vi "EOL CAN_Start CAN.vi"(8 "error in (no error)":errorcluster, 11 "CAN Interface":refnum<k21>="CAN1") -> (0 "error out":errorcluster, 1 "Tester Write Session out":refnum<k21>, 2 "Read Session out":refnum<k21>, 3 "DSC Write Session out":refnum<k21>, 4 "time out session out":refnum<k21>)   [LabVIEW 2018]
uses:
  <vilib>/xnet/xnet.llb/XNET CAN Comm State.ctl
  <vilib>/xnet/xnet.llb/XNET Control Scope.ctl
  <vilib>/xnet/xnet.llb/XNET Frame CAN.ctl
  <vilib>/xnet/xnet.llb/XNET Frame Type CAN.ctl
  <vilib>/xnet/xnet.llb/XNET Create Session (Frame Input Queued).vi
  <vilib>/xnet/xnet.llb/XNET Create Session (Frame Output Single-point).vi
  <vilib>/xnet/xnet.llb/XNET Write (Frame CAN).vi
  <vilib>/xnet/xnet.llb/XNET Read (State CAN Comm).vi
  <vilib>/xnet/xnet.llb/XNET Wait (Interface Communicating).vi
  <resource>/objmgr/xnet.rc
panel:
  out "CAN:I/O Mode":u32(ring) items=["CAN 2.0", "CAN FD", "CAN FD+BRS"]
  out "Protocol":u32(ring) items=["CAN", "FlexRay", "LIN"]
  out "CAN:Transceiver Capability":u32(ring) items=["HS"=0, "LS"=1, "XS"=3, "XS (HS/LS)"=4]
  out "Interface:CAN:Transceiver State 3":u32(ring) items=["Normal", "Sleep", "Single Wire Wakeup", "Single Wire High-Speed"]
  out "Interface:CAN:Transceiver State 2":u32(ring) items=["Normal", "Sleep", "Single Wire Wakeup", "Single Wire High-Speed"]
  out "Interface:CAN:Transceiver State":u32(ring) items=["Normal", "Sleep", "Single Wire Wakeup", "Single Wire High-Speed"]
  out "PDUs":refnum<k21>[](array[refnum])
  out "Frames":refnum<k21>[](array[refnum])
  out "ECUs":refnum<k21>[](array[refnum])
  out "Database":refnum<k21>
  out "Configuration Status":i32
  out "CAN:Termination Capability":u32(ring) items=["No", "Yes"]
  out "Array":T1[](array[typedef]) items=["Error Active", "Error Passive", "Bus Off", "Init"]
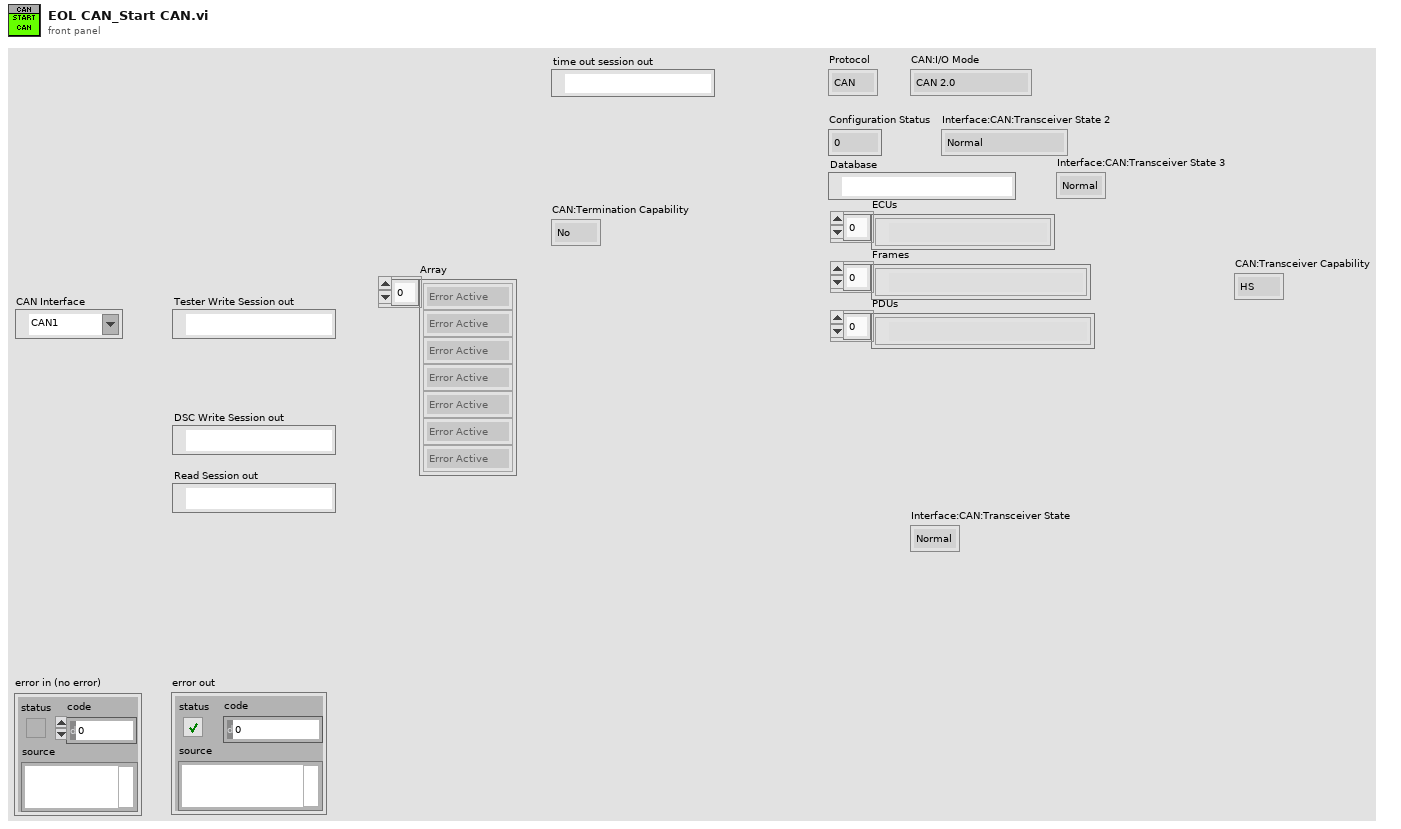
[diagram p1: front panel]
types:
  T1 = typedef "XNET CAN Comm State.ctl" = u8
  T2 = typedef "XNET Control Scope.ctl" = u32
  T3 = cluster{"Comment":string, "Default Payload":u8[], "Identifier":u32, "Name (Short)":string, "Payload Length":u32, "PDU_Mapping":cluster{"PDU":string, "Start Bit":u32, "Update Bit":i32}[], "CAN:Extended Identifier?":bool, "CAN:Timing Type":u32, "CAN:Transmit Time":dbl, "CAN:I/O Mode":u32}
  T4 = typedef "XNET Frame CAN.ctl" = cluster{"timestamp":timestamp, "payload":u8[], "identifier":u32, "type":T5, "extended?":bool, "echo?":bool}
  T5 = typedef "XNET Frame Type CAN.ctl" = u8
  T6 = typedef "XNET CAN Comm.ctl" = cluster{"fault code":i32, "fault?":bool, "communication state":T1, "last error":T7, "receive error counter":u8, "transmit error counter":u8, "transceiver error?":bool, "sleep?":bool}
  T7 = typedef "XNET CAN Last Err.ctl" = u8
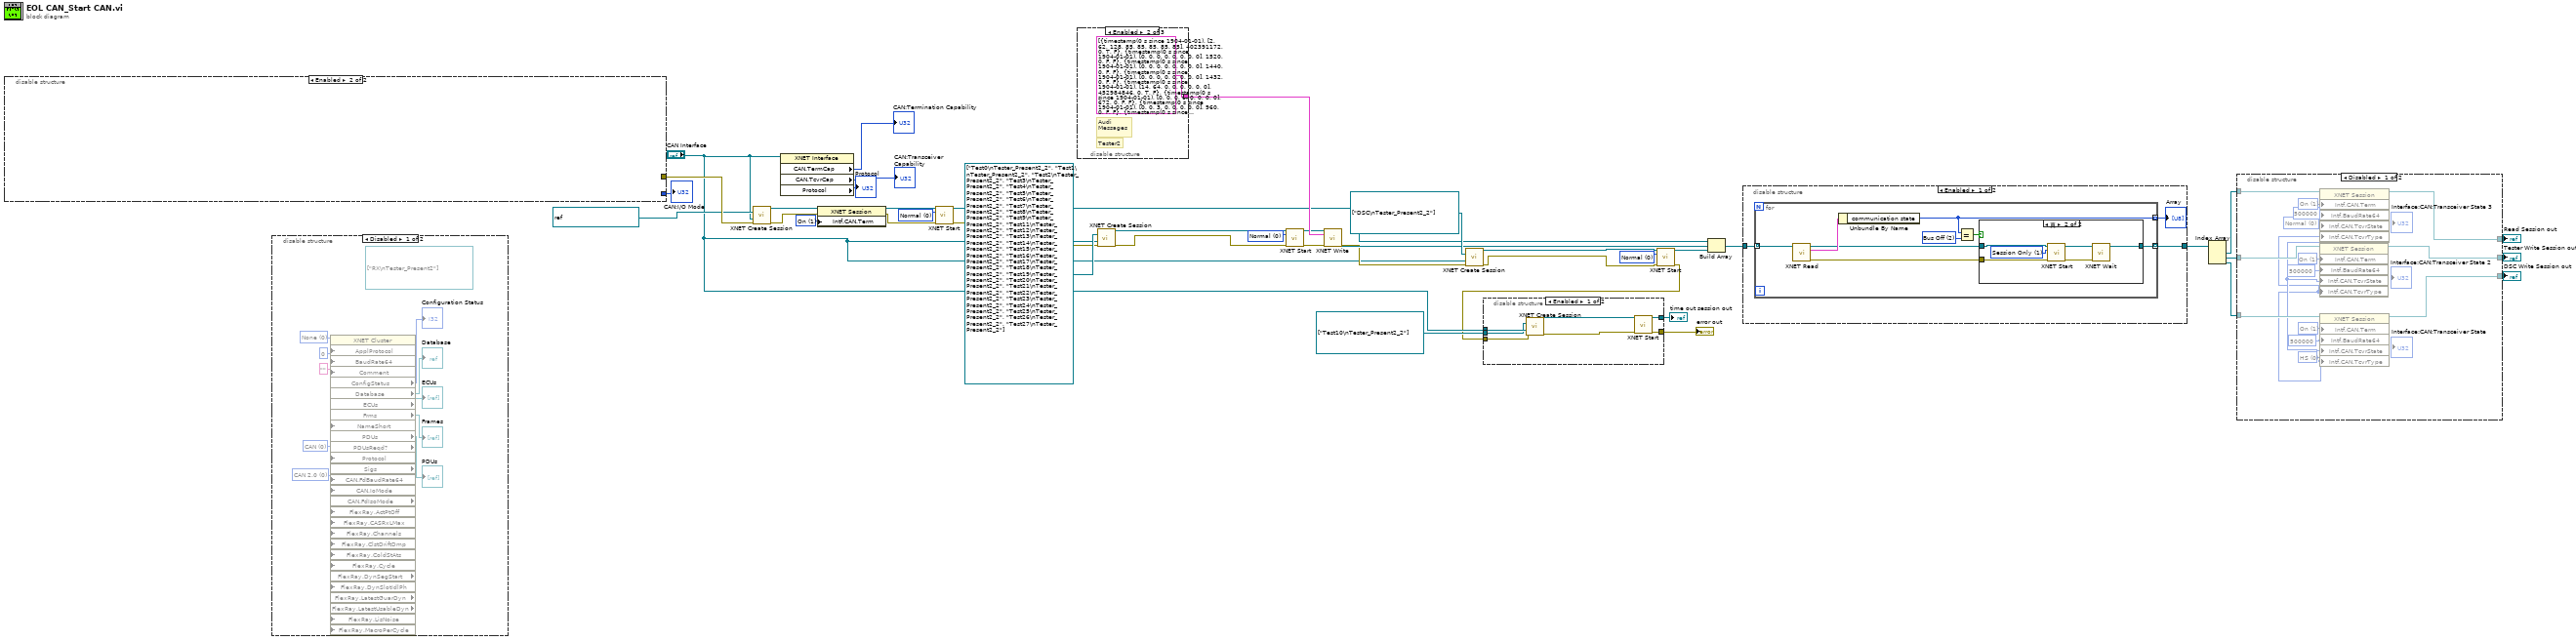
[diagram p0: block diagram]
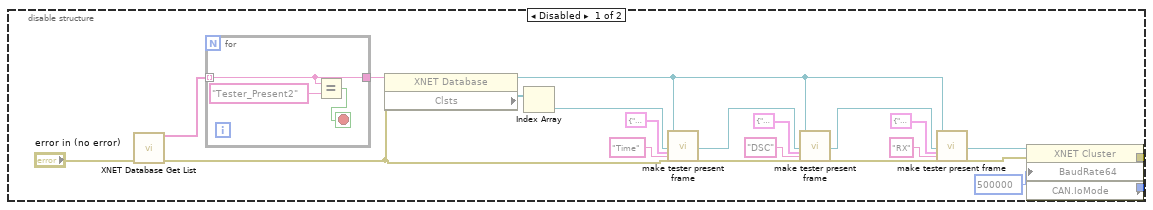
[diagram p2: hidden frame]
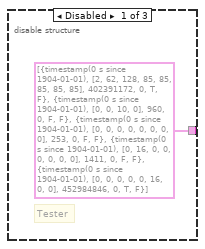
[diagram p8: hidden frame]
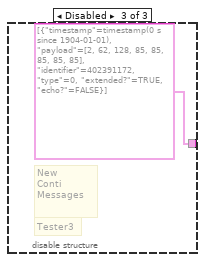
[diagram p9: hidden frame]
diagram:
  w7 = u32 1 items=["Off", "On"] ("Interface:CAN:Termination")
  w26 = T2 0 items=["Normal", "Session Only", "Interface Only", "Session Only Blocking"] ("scope (normal)")
  w27 = T2 0 items=["Normal", "Session Only", "Interface Only", "Session Only Blocking"] ("scope (normal)")
  w28 = T2 0 items=["Normal", "Session Only", "Interface Only", "Session Only Blocking"] ("scope (normal)")
  n1 = disable-structure shown="Enabled" {
    disable-tunnel: [w61 _] -> w41
    disable-tunnel: [w42 _] -> w11
    frame Disabled {
      n2 = call <vilib>:"XNET Database Get List.vi"("error in (no error)"="error in (no error)") -> ("array of alias"=w51:string[], "error out"=w47:errorcluster)  [unwired: 12 in, 1 out]
      n3 = for {
        tunnel: w51 -> [w64] mode=indexing
        tunnel: [w64] -> w50
        stop <- w65 stop-if-true
        n4 = Equal?(x=w64, y="Tester_Present2") -> (x = y?=w65:bool)
      }
      n5 = property class="XNET Database"(reference=w50, error in=w47) -> (reference out=w43:refnum<k21>, "Clsts"=w62:refnum<k21>[])  [unwired: 1 out]
      n6 = Index Array(array=w62) -> (element=w45:refnum<k21>)  [unwired: 1 in]
      n7 = call <userlib>:"make tester present frame.vi"("Cluster::"=w45, "New Frame Properties"=T3 {"Comment"="DSC", "Default Payload"=[0, 0, 0, 0, 0, 0, 0, 0], "Identifier"=1714, "Name (Short)"="Time", "Payload Length"=8, "PDU_Mapping"=[], "CAN:Extended Identifier?"=FALSE, "CAN:Timing Type"=0, "CAN:Transmit Time"=0.001, "CAN:I/O Mode"=0}, "frame name"="Time", "error in (no error)"=w47, "database in"=w43) -> ("target cluster out"=w44:refnum<k21>, "error out"=w46:errorcluster)  [unwired: 21 in]
      n8 = call <userlib>:"make tester present frame.vi"("Cluster::"=w44, "New Frame Properties"=T3 {"Comment"="DSC", "Default Payload"=[0, 0, 0, 0, 0, 0, 0, 0], "Identifier"=402391172, "Name (Short)"="DSC", "Payload Length"=8, "PDU_Mapping"=[], "CAN:Extended Identifier?"=TRUE, "CAN:Timing Type"=1, "CAN:Transmit Time"=0.001, "CAN:I/O Mode"=0}, "frame name"="DSC", "error in (no error)"=w46, "database in"=w43) -> ("target cluster out"=w60:refnum<k21>, "error out"=w59:errorcluster)  [unwired: 21 in]
      n9 = call <userlib>:"make tester present frame.vi"("Cluster::"=w60, "New Frame Properties"=T3 {"Comment"="RX", "Default Payload"=[0, 127, 0, 0, 0, 0, 0, 0], "Identifier"=402522244, "Name (Short)"="RX", "Payload Length"=8, "PDU_Mapping"=[], "CAN:Extended Identifier?"=TRUE, "CAN:Timing Type"=1, "CAN:Transmit Time"=0.001, "CAN:I/O Mode"=0}, "frame name"="RX", "error in (no error)"=w59, "database in"=w43) -> ("target cluster out"=w53:refnum<k21>, "error out"=w52:errorcluster)  [unwired: 21 in]
      n10 = property class="XNET Cluster"(reference=w53, error in=w52, "BaudRate64"=u64 500000 ("64bit Baud Rate")) -> (error out=w61:errorcluster, "CAN.IoMode"=w42:u32)  [unwired: 1 out]
    }
    frame Enabled {
    }
  }
  "CAN:I/O Mode" <- w11
  n11 = disable-structure shown="Disabled" {
    frame Disabled {
      w67 = u32 0 items=["CAN 2.0", "CAN FD", "CAN FD+BRS"] ("CAN:I/O Mode")
      w68 = u32 0 items=["CAN", "FlexRay", "LIN"] ("Protocol")
      w76 = u32 0 items=["None", "J1939"] ("Application Protocol")
      (unwired) refnum<k21>[] ["RX\nTester_Present2"]
      n12 = property class="XNET Cluster" props=["ApplProtocol", "BaudRate64", "Comment", "ConfigStatus", "Database", "ECUs", "Frms", "NameShort", "PDUs", "PDUsReqd?", "Protocol", "Sigs", "CAN.FdBaudRate64", "CAN.IoMode", "CAN.FdIsoMode", "FlexRay.ActPtOff", "FlexRay.CASRxLMax", "FlexRay.Channels", "FlexRay.ClstDriftDmp", "FlexRay.ColdStAts", "FlexRay.Cycle", "FlexRay.DynSegStart", "FlexRay.DynSlotIdlPh", "FlexRay.LatestGuarDyn", "FlexRay.LatestUsableDyn", "FlexRay.LisNoise", "FlexRay.MacroPerCycle"]("ApplProtocol"=w76, "BaudRate64"=u64 0 ("64bit Baud Rate"), "Comment"="", "Protocol"=w68, "CAN.IoMode"=w67) -> ("ConfigStatus"=→"Configuration Status":i32, "Database"=→"Database":refnum<k21>, "ECUs"=→"ECUs":refnum<k21>[], "Frms"=→"Frames":refnum<k21>[], "PDUs"=→"PDUs":refnum<k21>[])  [unwired: 13 in, 8 out]
    }
    frame Enabled {
    }
  }
  n13 = call-poly <vilib>:"XNET Create Session.vi"("frame"=refnum<k21> "RX\nTester_Present2_2" ("XNET Frame"), "interface"="CAN Interface", "error in (no error)"=w41) -> ("session out"=w10:refnum<k21>, "error out"=w8:errorcluster)  [unwired: 11 in]
  n14 = property class="XNET Interface"(reference="CAN Interface") -> ("CAN.TermCap"=→"CAN:Termination Capability":u32, "CAN.TcvrCap"=→"CAN:Transceiver Capability":u32, "Protocol"=→"Protocol":u32)  [unwired: 1 in, 2 out]
  n15 = property class="XNET Session"(reference=w10, error in=w8, "Intf.CAN.Term"=w7) -> (reference out=w9:refnum<k21>, error out=w6:errorcluster)
  n16 = call <vilib>:"XNET Start.vi"("session in"=w9, "scope (normal)"=w28, "error in (no error)"=w6) -> ("session out"=w35:refnum<k21>, "error out"=w30:errorcluster)  [unwired: 11 in]
  n17 = disable-structure shown="Enabled" {
    disable-tunnel: [T4[] [{"timestamp"=timestamp(0 s since 1904-01-01), "payload"=[2, 62, 128, 85, 85, 85, 85, 85], "identifier"=402391172, "type"=0, "extended?"=TRUE, "echo?"=FALSE}, {"timestamp"=timestamp(0 s since 1904-01-01), "payload"=[0, 0, 10, 0], "identifier"=960, "type"=0, "extended?"=FALSE, "echo?"=FALSE}, {"timestamp"=timestamp(0 s since 1904-01-01), "payload"=[0, 0, 0, 0, 0, 0, 0, 0], "identifier"=253, "type"=0, "extended?"=FALSE, "echo?"=FALSE}, {"timestamp"=timestamp(0 s since 1904-01-01), "payload"=[0, 16, 0, 0, 0, 0, 0, 0], "identifier"=1411, "type"=0, "extended?"=FALSE, "echo?"=FALSE}, {"timestamp"=timestamp(0 s since 1904-01-01), "payload"=[0, 0, 0, 0, 0, 16, 0, 0], "identifier"=452984846, "type"=0, "extended?"=TRUE, "echo?"=FALSE}] ("data") T4[] [{"timestamp"=timestamp(0 s since 1904-01-01), "payload"=[2, 62, 128, 85, 85, 85, 85, 85], "identifier"=402391172, "type"=0, "extended?"=TRUE, "echo?"=FALSE}, {"timestamp"=timestamp(0 s since 1904-01-01), "payload"=[0, 0, 0, 0, 0, 0, 0, 0], "identifier"=1520, "type"=0, "extended?"=FALSE, "echo?"=FALSE}, {"timestamp"=timestamp(0 s since 1904-01-01), "payload"=[0, 0, 0, 0, 0, 0, 0, 0], "identifier"=1440, "type"=0, "extended?"=FALSE, "echo?"=FALSE}, {"timestamp"=timestamp(0 s since 1904-01-01), "payload"=[0, 0, 0, 0, 0, 0, 0, 0], "identifier"=1432, "type"=0, "extended?"=FALSE, "echo?"=FALSE}, {"timestamp"=timestamp(0 s since 1904-01-01), "payload"=[14, 64, 0, 0, 0, 0, 0, 0], "identifier"=452984846, "type"=0, "extended?"=TRUE, "echo?"=FALSE}, {"timestamp"=timestamp(0 s since 1904-01-01), "payload"=[0, 0, 0, 0, 0, 0, 0, 0], "identifier"=672, "type"=0, "extended?"=FALSE, "echo?"=FALSE}, {"timestamp"=timestamp(0 s since 1904-01-01), "payload"=[0, 0, 3, 0, 0, 0, 0, 0], "identifier"=960, "type"=0, "extended?"=FALSE, "echo?"=FALSE}, {"timestamp"=timestamp(0 s since 1904-01-01), "payload"=[0, 0, 0, 0, 0, 0, 0, 0], "identifier"=1716, "type"=0, "extended?"=FALSE, "echo?"=FALSE}, {"timestamp"=timestamp(0 s since 1904-01-01), "payload"=[0, 16, 0, 0, 0, 0, 0, 0], "identifier"=1411, "type"=0, "extended?"=FALSE, "echo?"=FALSE}, {"timestamp"=timestamp(0 s since 1904-01-01), "payload"=[139, 64, 0, 0, 0, 0, 0, 0], "identifier"=452984971, "type"=0, "extended?"=TRUE, "echo?"=FALSE}, {"timestamp"=timestamp(0 s since 1904-01-01), "payload"=[0, 0, 0, 0, 0, 0, 0, 0], "identifier"=253, "type"=0, "extended?"=FALSE, "echo?"=FALSE}, {"timestamp"=timestamp(0 s since 1904-01-01), "payload"=[0, 0, 0, 0, 0, 0, 0, 0], "identifier"=508, "type"=0, "extended?"=FALSE, "echo?"=FALSE}, {"timestamp"=timestamp(0 s since 1904-01-01), "payload"=[0, 0, 0, 0, 150, 0, 0, 0], "identifier"=1646, "type"=0, "extended?"=FALSE, "echo?"=FALSE}, {"timestamp"=timestamp(0 s since 1904-01-01), "payload"=[0, 0, 0, 0, 0, 0, 0, 150], "identifier"=1719, "type"=0, "extended?"=FALSE, "echo?"=FALSE}, {"timestamp"=timestamp(0 s since 1904-01-01), "payload"=[0, 0, 4, 0, 0, 0, 0, 0], "identifier"=958, "type"=0, "extended?"=FALSE, "echo?"=FALSE}, {"timestamp"=timestamp(0 s since 1904-01-01), "payload"=[0, 0, 0, 0, 0, 0, 0, 0], "identifier"=1635, "type"=0, "extended?"=FALSE, "echo?"=FALSE}, {"timestamp"=timestamp(0 s since 1904-01-01), "payload"=[0, 0, 0, 0, 0, 0, 0, 0], "identifier"=319, "type"=0, "extended?"=FALSE, "echo?"=FALSE}, {"timestamp"=timestamp(0 s since 1904-01-01), "payload"=[0, 0, 0, 0, 0, 0, 0, 0], "identifier"=1616, "type"=0, "extended?"=FALSE, "echo?"=FALSE}, {"timestamp"=timestamp(0 s since 1904-01-01), "payload"=[0, 12, 0, 0, 0, 0, 0, 0], "identifier"=1413, "type"=0, "extended?"=FALSE, "echo?"=FALSE}, {"timestamp"=timestamp(0 s since 1904-01-01), "payload"=[0, 0, 0, 0, 0, 0, 0, 0], "identifier"=1462, "type"=0, "extended?"=FALSE, "echo?"=FALSE}, {"timestamp"=timestamp(0 s since 1904-01-01), "payload"=[16, 64, 0, 0, 0, 16, 0, 0], "identifier"=452984848, "type"=0, "extended?"=TRUE, "echo?"=FALSE}, {"timestamp"=timestamp(0 s since 1904-01-01), "payload"=[0, 0, 0, 0, 0, 0, 0, 0], "identifier"=976, "type"=0, "extended?"=FALSE, "echo?"=FALSE}, {"timestamp"=timestamp(0 s since 1904-01-01), "payload"=[0, 0, 0, 0, 0, 0, 0, 0], "identifier"=974, "type"=0, "extended?"=FALSE, "echo?"=FALSE}, {"timestamp"=timestamp(0 s since 1904-01-01), "payload"=[74, 64, 0, 0, 0, 0, 0, 0], "identifier"=452984906, "type"=0, "extended?"=TRUE, "echo?"=FALSE}, {"timestamp"=timestamp(0 s since 1904-01-01), "payload"=[0, 0, 0, 0, 0, 0, 0, 0], "identifier"=977, "type"=0, "extended?"=FALSE, "echo?"=FALSE}, {"timestamp"=timestamp(0 s since 1904-01-01), "payload"=[0, 0, 0, 0, 0, 0, 0, 0], "identifier"=975, "type"=0, "extended?"=FALSE, "echo?"=FALSE}, {"timestamp"=timestamp(0 s since 1904-01-01), "payload"=[75, 64, 0, 0, 0, 0, 0, 0], "identifier"=452984907, "type"=0, "extended?"=TRUE, "echo?"=FALSE}] ("Array 3") T4[] [{"timestamp"=timestamp(0 s since 1904-01-01), "payload"=[2, 62, 128, 85, 85, 85, 85, 85], "identifier"=402391172, "type"=0, "extended?"=TRUE, "echo?"=FALSE}] ("data")] -> w40
    frame Disabled {
      # "Tester"
    }
    frame Enabled {
      # "Tester2"
      # "Audi\nMessages"
    }
    frame Disabled {
      # "Tester3"
      # "New\nConti\nMessages"
    }
  }
  n18 = call-poly <vilib>:"XNET Create Session.vi"("frame list"=refnum<k21>[] ["Test0\nTester_Present2_2", "Test1\nTester_Present2_2", "Test2\nTester_Present2_2", "Test3\nTester_Present2_2", "Test4\nTester_Present2_2", "Test5\nTester_Present2_2", "Test6\nTester_Present2_2", "Test7\nTester_Present2_2", "Test8\nTester_Present2_2", "Test9\nTester_Present2_2", "Test11\nTester_Present2_2", "Test12\nTester_Present2_2", "Test13\nTester_Present2_2", "Test14\nTester_Present2_2", "Test15\nTester_Present2_2", "Test16\nTester_Present2_2", "Test17\nTester_Present2_2", "Test18\nTester_Present2_2", "Test19\nTester_Present2_2", "Test20\nTester_Present2_2", "Test21\nTester_Present2_2", "Test22\nTester_Present2_2", "Test23\nTester_Present2_2", "Test24\nTester_Present2_2", "Test25\nTester_Present2_2", "Test26\nTester_Present2_2", "Test27\nTester_Present2_2"] ("Frames"), "interface"="CAN Interface", "error in (no error)"=w30) -> ("session out"=w23:refnum<k21>, "error out"=w24:errorcluster)  [unwired: 11 in]
  n19 = call <vilib>:"XNET Start.vi"("session in"=w23, "scope (normal)"=w27, "error in (no error)"=w24) -> ("session out"=w39:refnum<k21>, "error out"=w38:errorcluster)  [unwired: 11 in]
  n20 = call-poly <vilib>:"XNET Write.vi"("session in"=w39, "data"=w40, "error in (no error)"=w38) -> ("session out"=w34:refnum<k21>, "error out"=w29:errorcluster)  [unwired: 11 in]
  n21 = call-poly <vilib>:"XNET Create Session.vi"("frame list"=refnum<k21>[] ["DSC\nTester_Present2_2"] ("Frames"), "interface"="CAN Interface", "error in (no error)"=w29) -> ("session out"=w22:refnum<k21>, "error out"=w21:errorcluster)  [unwired: 11 in]
  n22 = call <vilib>:"XNET Start.vi"("session in"=w22, "scope (normal)"=w26, "error in (no error)"=w21) -> ("session out"=w33:refnum<k21>, "error out"=w1:errorcluster)  [unwired: 11 in]
  n23 = disable-structure shown="Enabled" {
    disable-tunnel: "CAN Interface" -> [w86 _]
    disable-tunnel: [w85 _] -> w3
    disable-tunnel: [w84 _] -> w2
    disable-tunnel: refnum<k21>[] ["Test10\nTester_Present2_2"] ("Frames") -> [w83 _]
    disable-tunnel: w1 -> [w80 _]
    frame Enabled {
      n24 = call-poly <vilib>:"XNET Create Session.vi"("frame list"=w83, "interface"=w86, "error in (no error)"=w80) -> ("session out"=w82:refnum<k21>, "error out"=w81:errorcluster)  [unwired: 11 in]
      n25 = call <vilib>:"XNET Start.vi"("session in"=w82, "error in (no error)"=w81) -> ("session out"=w85:refnum<k21>, "error out"=w84:errorcluster)  [unwired: 12 in]
    }
    frame Disabled {
    }
  }
  "error out" <- w2
  "time out session out" <- w3
  n26 = Build Array(w35, w34, w33) -> (w32:refnum<k21>[])
  n27 = disable-structure shown="Enabled" {
    disable-tunnel: w32 -> [w89 w105]
    disable-tunnel: [w87 w105] -> w31
    frame Enabled {
      n28 = for {
        tunnel: w89 -> [w96] mode=indexing
        tunnel: [w91] -> w88 mode=indexing
        tunnel: [w90] -> w87 mode=indexing
        w95 = T1 2 items=["Error Active", "Error Passive", "Bus Off", "Init"] ("y")
        n29 = call-poly <vilib>:"XNET Read.vi"("session in"=w96) -> ("session out"=w93:refnum<k21>, "CAN comm"=w97:T6, "error out"=w92:errorcluster)  [unwired: 12 in]
        n30 = Unbundle By Name(w97) -> ("communication state"=w91:T1)
        n31 = Equal?(x=w91, y=w95) -> (x = y?=w94:bool)
        n32 = case shown="真" w94 {
          tunnel: w93 -> [w98 w104]
          tunnel: w92 -> [_ w102]
          tunnel: [w98 w99] -> w90
          frame False {
          }
          frame True {
            w100 = T2 1 items=["Normal", "Session Only", "Interface Only", "Session Only Blocking"] ("scope (normal)")
            n33 = call <vilib>:"XNET Start.vi"("session in"=w104, "scope (normal)"=w100, "error in (no error)"=w102) -> ("session out"=w103:refnum<k21>, "error out"=w101:errorcluster)  [unwired: 11 in]
            n34 = call-poly <vilib>:"XNET Wait.vi"("session in"=w103, "error in (no error)"=w101) -> ("session out"=w99:refnum<k21>)  [unwired: 12 in, 1 out]
          }
        }
      }
      "Array" <- w88
    }
    frame Disabled {
    }
  }
  n35 = Index Array(array=w31) -> (element #1=w19:refnum<k21>, element #2=w17:refnum<k21>, element #3=w15:refnum<k21>)  [unwired: 3 in]
  n36 = disable-structure shown="Disabled" {
    disable-tunnel: w19 -> [w118 w122]
    disable-tunnel: [w117 w122] -> w18
    disable-tunnel: w17 -> [w114 w121]
    disable-tunnel: [w113 w121] -> w16
    disable-tunnel: w15 -> [w112 w120]
    disable-tunnel: [w111 w120] -> w14
    frame Disabled {
      w106 = u32 0 items=["HS", "LS", "SW", "Ext", "Disc"] ("Interface:CAN:Transceiver Type")
      w107 = u32 0 items=["Normal", "Sleep", "Single Wire Wakeup", "Single Wire High-Speed"] ("Interface:CAN:Transceiver State")
      w115 = u32 1 items=["Off", "On"] ("Interface:CAN:Termination")
      w116 = u32 1 items=["Off", "On"] ("Interface:CAN:Termination")
      w119 = u32 1 items=["Off", "On"] ("Interface:CAN:Termination")
      n37 = property class="XNET Session"(reference=w114, "Intf.CAN.Term"=w116, "Intf.BaudRate64"=u64 500000 ("Interface:64bit Baud Rate"), "Intf.CAN.TcvrState"=w107, "Intf.CAN.TcvrType"=w106) -> (reference out=w113:refnum<k21>)  [unwired: 1 in, 1 out]
      n38 = property class="XNET Session"(reference=w118, "Intf.CAN.Term"=w119, "Intf.BaudRate64"=u64 500000 ("Interface:64bit Baud Rate"), "Intf.CAN.TcvrState"=w107, "Intf.CAN.TcvrType"=w106) -> (reference out=w117:refnum<k21>)  [unwired: 1 in, 1 out]
      n39 = property class="XNET Session"(reference=w112, "Intf.CAN.Term"=w115, "Intf.BaudRate64"=u64 500000 ("Interface:64bit Baud Rate"), "Intf.CAN.TcvrState"=w107, "Intf.CAN.TcvrType"=w106) -> (reference out=w111:refnum<k21>)  [unwired: 1 in, 1 out]
    }
    frame Enabled {
    }
  }
  "Tester Write Session out" <- w16
  "Read Session out" <- w18
  "DSC Write Session out" <- w14
